vi "NoiseOutput_PXIe-7962R.vi"() -> ()   [LabVIEW 2012]
uses:
  <vilib>/Platform/TimedLoop/XDataNode/timing_clust.ctl
  <vilib>/Platform/TimedLoop/XDataNode/nitl_modes.ctl
  <vilib>/Platform/TimedLoop/XDataNode/wakeup.ctl
  <vilib>/rvi/Emulation/niFpgaSctlEmulationRegisterWithScheduler.vi
  <vilib>/rvi/Emulation/niFpgaSctlEmulationGlobalWrite.vi
  <vilib>/rvi/eio/common/nirviEmuTemplateMethod_errors.vi
  <vilib>/rvi/interface/RandomDataEmulation/nirviRandomDataFPGAFIFO.vi
  <vilib>/rvi/interface/RandomDataEmulation/niFpgaRandomDataHandleErrors.vi
  <vilib>/rvi/Emulation/niFpgaSctlEmulationScheduler.vi
  <vilib>/Platform/TimedLoop/XDataNode/XDataNode.xnode
  <vilib>/eio/EIONode/EIONode.xnode
  <vilib>/rvi/DataTransferAndStorage/Container/XNode/niFpgaContainer.xnode
  <vilib>/rvi/interface/RandomDataEmulation/nirviRandomDataFpgaReadWriteTemplate.vi
  <vilib>/Platform/TimedLoop/XDataNode/XDNodeRunTimeDep.lvlib
panel:
  in  "Requested pixels A2":u32=100000 caption="Requested pixels"
  in  "Samples per pixel A1":u32
  out "Acquiring":bool
  out "ToHostA2Ch2Overflow":bool
  out "ToHostA2Ch1Overflow":bool
  out "ToHostA1Ch2Overflow":bool
  out "ToHostA1Ch1Overflow":bool
  in  "Wait for trigger":bool
  in  "Acquire":bool
  in  "Acquire continuously":bool=TRUE
  in  "Requested pixels A1":u32=100000 caption="Requested pixels"
  in  "Samples per line A2":u32
  in  "Samples per line A1":u32
  in  "Samples per pixel A2":u32
  in  "Quit":bool
  # "Acquisition control"
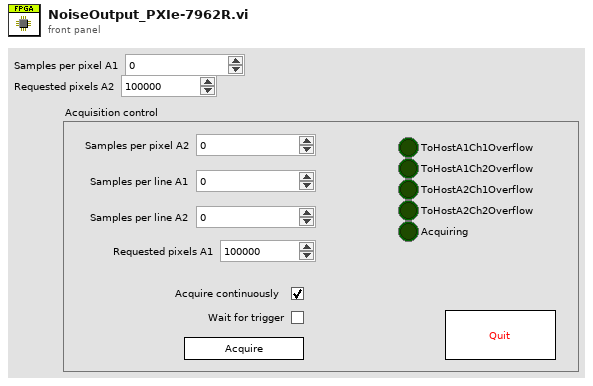
[diagram p1: front panel]
types:
  T1 = typedef "XDNodeRunTimeDep.lvlib/timing_clust.ctl" = cluster{"Expected End [f-1]":u64, "Actual End [f-1]":u64, "Finished Late? [f-1]":bool, "Expected End [i-1]":u64, "Actual End [i-1]":u64, "Finished Late? [i-1]":bool, "Expected Start [i]":u64, "Actual Start [i]":u64, "Expected Start [f]":u64, "Actual Start [f]":u64, "Source Name":string, "Structure Name":string, "Period":i64, "Deadline":i64, "Offset":i64, "Start":i64, "Priority":i32, "Timeout":i32, "Mode":T2, "Wakeup Reason":T3, "Error":errorcluster, "Source Type":string, "Secondary Source Type":string, "Global End Time":u64, "Global Start Time":u64, "Frame Duration":u64, "Iteration Duration":u64, "Assigned CPU":i32, "I/O Scan Engine Mode":u32}
  T2 = typedef "XDNodeRunTimeDep.lvlib/nitl_modes.ctl" = enum32{"No Change", "Process missed periods, maintain original phase", "Discard missed periods, maintain original phase", "Process missed periods, ignore original phase", "Discard missed periods, ignore original phase"}
  T3 = typedef "XDNodeRunTimeDep.lvlib/wakeup.ctl" = enum32{"Normal", "Aborted", "Asynchronous wakeup", "Timing source error", "Timed loop error", "Timeout"}
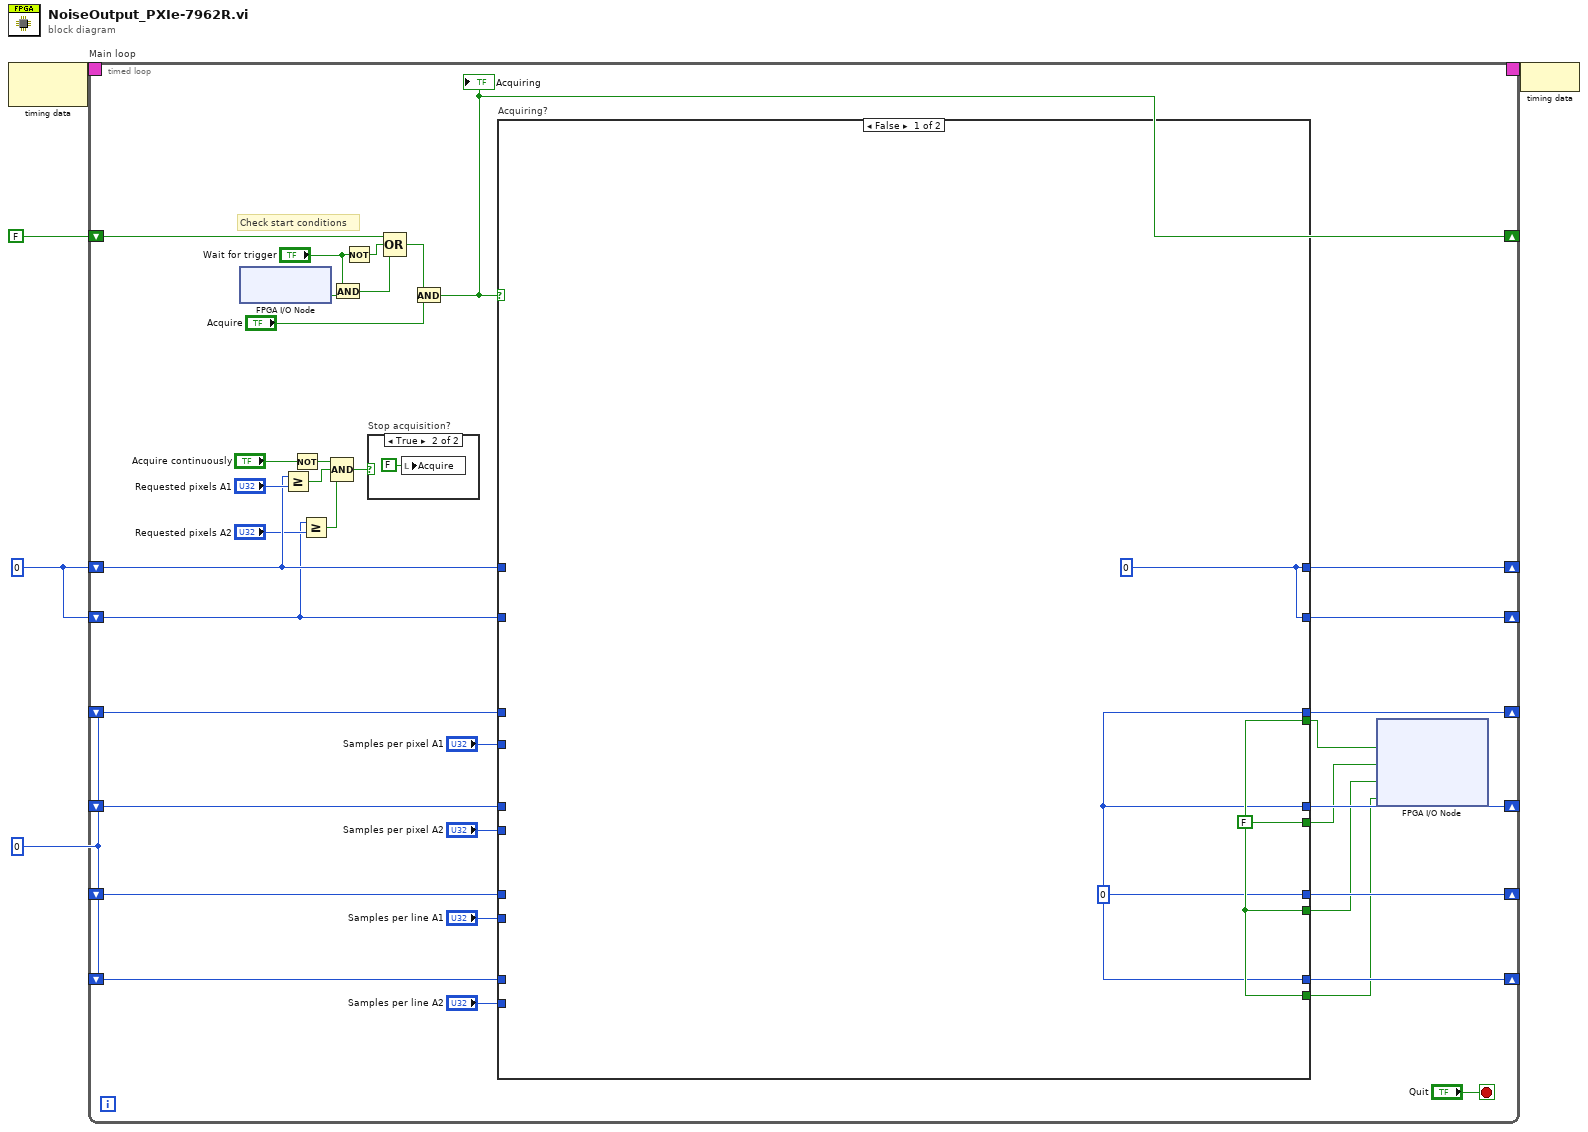
[diagram p0: block diagram]
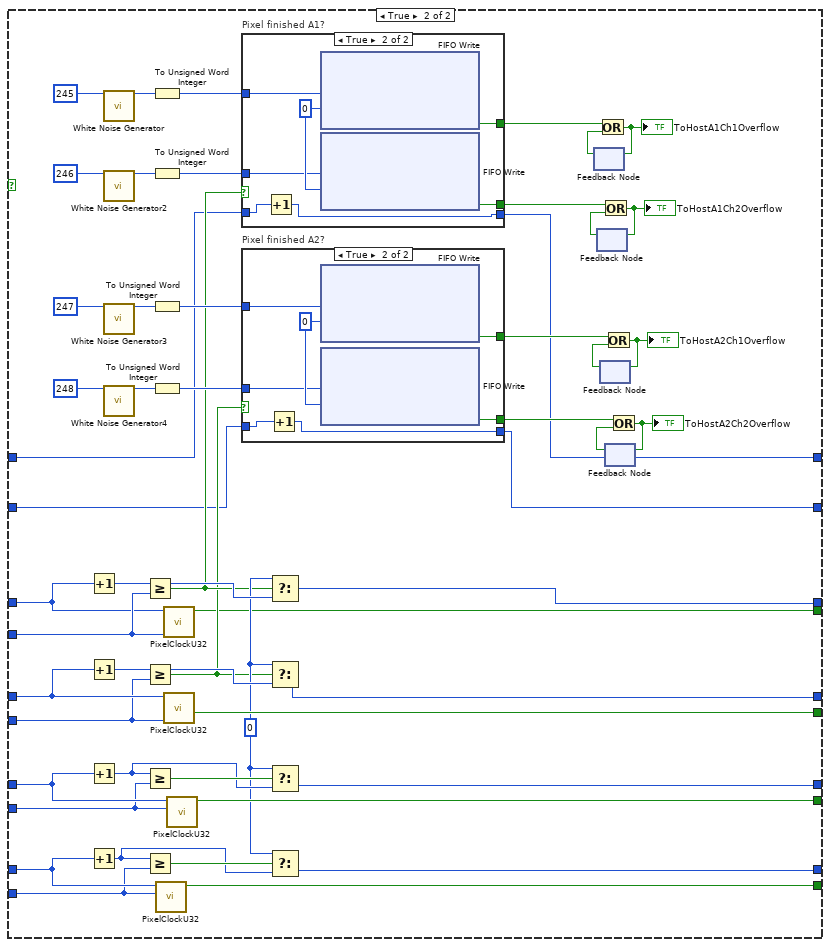
[diagram p3: hidden frame]
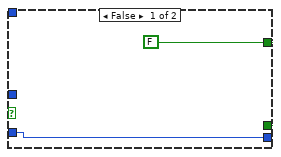
[diagram p4: hidden frame]
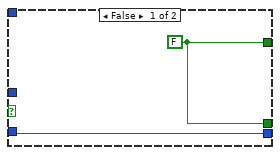
[diagram p5: hidden frame]
diagram:
  w1 = u32 0
  w2 = u32 0 ("Cycle counter out")
  n1 = node-c288() -> (w5:T1)  [unwired: 1 in]
  n2 = timed-loop "Main loop" {
    timing: w5 -> [_]
    timing-out: [_] -> w4
    shift-right: [w40] -> _
    shift-left: w2 -> [w39]
    shift-right: [w37] -> _
    shift-left: w2 -> [w36]
    shift-right: [w34] -> _
    shift-left: w2 -> [w33]
    shift-right: [w17] -> _
    shift-left: FALSE -> [w20]
    shift-right: [w18] -> _
    shift-left: w1 -> [w19]
    shift-right: [w6] -> _
    shift-left: w2 -> [w16]
    shift-right: [w14] -> _
    shift-left: w1 -> [w12]
    stop <- "Quit" stop-if-true
    # "Check start conditions"
    n3 = xnode "FPGA I/O Node"() -> ("TriggerIn"=w26:bool)  [unwired: 1 in, 1 out]
    n4 = Greater Or Equal?(x=w19, y="Requested pixels A1") -> (x >= y?=w28:bool)
    n5 = Not(x="Acquire continuously") -> (.not. x?=w29:bool)
    n6 = Greater Or Equal?(x=w12, y="Requested pixels A2") -> (x >= y?=w11:bool)
    n7 = Compound Arithmetic op=AND(w29, w28, w11) -> (w27:bool)
    n8 = And(x="Wait for trigger", y=w26) -> (x .and. y?=w23:bool)
    n9 = Not(x="Wait for trigger") -> (.not. x?=w24:bool)
    n10 = case "Stop acquisition?" shown="True" w27 {
      frame False {
      }
      frame True {
        n11 = local write "Acquire"(FALSE ("Acquire")) -> ()
      }
    }
    n12 = Compound Arithmetic op=OR(w20, w24, w23) -> (w22:bool)
    n13 = And(x=w22, y="Acquire") -> (x .and. y?=w17:bool)
    "Acquiring" <- w17
    n14 = case "Acquiring?" shown="False" w17 {
      tunnel: [w43 w89] -> w40
      tunnel: w39 -> [_ w97]
      tunnel: "Samples per pixel A2" -> [_ w96]
      tunnel: [w43 w88] -> w37
      tunnel: w36 -> [_ w92]
      tunnel: "Samples per line A1" -> [_ w91]
      tunnel: [w43 w83] -> w34
      tunnel: w33 -> [_ w85]
      tunnel: "Samples per line A2" -> [_ w84]
      tunnel: [w44 w98] -> w9
      tunnel: [w44 w90] -> w8
      tunnel: [w44 w82] -> w7
      tunnel: w19 -> [_ w51]
      tunnel: [w45 w48] -> w18
      tunnel: w16 -> [_ w55]
      tunnel: "Samples per pixel A1" -> [_ w56]
      tunnel: w12 -> [_ w50]
      tunnel: [w45 w49] -> w14
      tunnel: [w44 w47] -> w10
      tunnel: [w43 w46] -> w6
      frame False {
        w45 = u32 0 ("t")
        w43 = u32 0 ("t")
        w44 = FALSE
      }
      frame True {
        w54 = u32 0 ("t")
        n15 = Increment(x=w55) -> (x+1=w57:u32)
        n16 = Increment(x=w97) -> (x+1=w95:u32)
        n17 = Increment(x=w92) -> (x+1=w93:u32)
        n18 = Increment(x=w85) -> (x+1=w86:u32)
        n19 = call "White Noise Generator"("seed"=u32 245) -> ("white noise out"=w68:i16)  [unwired: 14 in]
        n20 = call "White Noise Generator2"("seed"=u32 246) -> ("white noise out"=w69:i16)  [unwired: 14 in]
        n21 = call "White Noise Generator3"("seed"=u32 247) -> ("white noise out"=w70:i16)  [unwired: 14 in]
        n22 = call "White Noise Generator4"("seed"=u32 248) -> ("white noise out"=w71:i16)  [unwired: 14 in]
        n23 = Greater Or Equal?(x=w57, y=w56) -> (x >= y?=w53:bool)
        n24 = Greater Or Equal?(x=w95, y=w96) -> (x >= y?=w52:bool)
        n25 = Greater Or Equal?(x=w93, y=w91) -> (x >= y?=w94:bool)
        n26 = Greater Or Equal?(x=w86, y=w84) -> (x >= y?=w87:bool)
        n27 = To Unsigned Word Integer(number=w68) -> (unsigned 16bit integer=w63:u16)
        n28 = To Unsigned Word Integer(number=w69) -> (unsigned 16bit integer=w62:u16)
        n29 = To Unsigned Word Integer(number=w70) -> (unsigned 16bit integer=w61:u16)
        n30 = To Unsigned Word Integer(number=w71) -> (unsigned 16bit integer=w60:u16)
        n31 = call "PixelClockU32.vi"("Samples per pixel"=w84, "Sample counter"=w85) -> ("Pixel clock"=w82:bool)  [unwired: 9 in]
        n32 = call "PixelClockU32.vi"("Samples per pixel"=w56, "Sample counter"=w55) -> ("Pixel clock"=w47:bool)  [unwired: 9 in]
        n33 = call "PixelClockU32.vi"("Samples per pixel"=w96, "Sample counter"=w97) -> ("Pixel clock"=w98:bool)  [unwired: 9 in]
        n34 = call "PixelClockU32.vi"("Samples per pixel"=w91, "Sample counter"=w92) -> ("Pixel clock"=w90:bool)  [unwired: 9 in]
        n35 = case "Pixel finished A1?" shown="True" w53 {
          tunnel: [w109 w115] -> w81
          tunnel: [w109 w114] -> w77
          tunnel: w63 -> [_ w113]
          tunnel: w62 -> [_ w112]
          tunnel: w51 -> [w108 w111]
          tunnel: [w108 w110] -> w48
          frame False {
            w109 = FALSE ("Timed Out?")
          }
          frame True {
            w116 = 0 ("Timeout")
            n36 = Increment(x=w111) -> (x+1=w110:u32)
            n37 = xnode "FIFO Write"("Element"=w113, "Timeout"=w116) -> ("Timed Out?"=w115:bool)  [unwired: 1 in, 1 out]
            n38 = xnode "FIFO Write"("Element"=w112, "Timeout"=w116) -> ("Timed Out?"=w114:bool)  [unwired: 1 in, 1 out]
          }
        }
        n39 = case "Pixel finished A2?" shown="True" w52 {
          tunnel: [w100 w106] -> w59
          tunnel: [w100 w105] -> w58
          tunnel: w61 -> [_ w104]
          tunnel: w60 -> [_ w103]
          tunnel: w50 -> [w99 w102]
          tunnel: [w99 w101] -> w49
          frame False {
            w100 = FALSE ("Timed Out?")
          }
          frame True {
            w107 = 0 ("Timeout")
            n40 = Increment(x=w102) -> (x+1=w101:u32)
            n41 = xnode "FIFO Write"("Element"=w104, "Timeout"=w107) -> ("Timed Out?"=w106:bool)  [unwired: 1 in, 1 out]
            n42 = xnode "FIFO Write"("Element"=w103, "Timeout"=w107) -> ("Timed Out?"=w105:bool)  [unwired: 1 in, 1 out]
          }
        }
        n43 = Select(t=w54, s=w53, f=w57) -> (s? t:f=w46:u32)
        n44 = Select(t=w54, s=w52, f=w95) -> (s? t:f=w89:u32)
        n45 = Select(t=w54, s=w94, f=w93) -> (s? t:f=w88:u32)
        n46 = Select(t=w54, s=w87, f=w86) -> (s? t:f=w83:u32)
        n47 = feedback #1() -> (w80:bool)  [unwired: 1 in]
        n48 = feedback #2() -> (w76:bool)  [unwired: 1 in]
        n49 = Or(x=w81, y=w80) -> (x .or. y?=w79:bool)
        "ToHostA1Ch1Overflow" <- w79
        n50 = feedback-in #1(w79) -> ()
        n51 = feedback #3() -> (w74:bool)  [unwired: 1 in]
        n52 = Or(x=w77, y=w76) -> (x .or. y?=w78:bool)
        "ToHostA1Ch2Overflow" <- w78
        n53 = feedback-in #2(w78) -> ()
        n54 = Or(x=w59, y=w74) -> (x .or. y?=w75:bool)
        "ToHostA2Ch1Overflow" <- w75
        n55 = feedback-in #3(w75) -> ()
        n56 = feedback #4() -> (w72:bool)  [unwired: 1 in]
        n57 = Or(x=w58, y=w72) -> (x .or. y?=w73:bool)
        "ToHostA2Ch2Overflow" <- w73
        n58 = feedback-in #4(w73) -> ()
      }
    }
    n59 = xnode "FPGA I/O Node"("PixelClockA1"=w10, "PixelClockA2"=w9, "LineClockA1"=w8, "LineClockA2"=w7) -> ()  [unwired: 4 in, 4 out]
  }
  n60 = node-c288(w4) -> ()
